vi "Set and Measure VSEC.vi"(4 "Header":string="HighVsec", 6 "Name":string, 7 "Position in":u32, 8 "error in (no error)":errorcluster, 9 "Measurement Wait Time":u32, 10 "Cree Comms in":refnum<class "Cree Communications.lvclass">, 11 "Calibration in":refnum<class "Calibration.lvclass">) -> (0 "error out":errorcluster, 2 "DSpic Measurement":dbl, 3 "Actual Measurement":dbl)   [LabVIEW 2015, in "Calibration.lvclass"]
uses:
  Calibration.lvclass
  Classes/Cree Communications/Class/Cree Communications.lvclass
  Classes/Cree Communications/Cree Comms Messages/Set Vsec/Set Vsec Reference.lvclass
  Classes/Cree Communications/Cree Comms Messages/CC Message/CC Message.lvclass/CC Message.ctl
  Test Class/Test Class.lvclass
  Classes/Cree Communications/Cree Comms Messages/CC Message/CC Message.lvclass
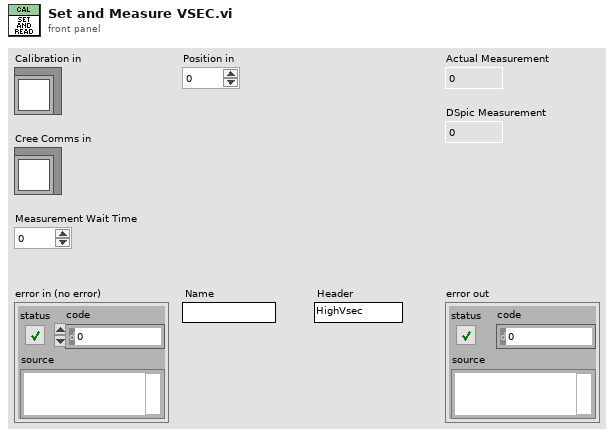
[diagram p1: front panel]
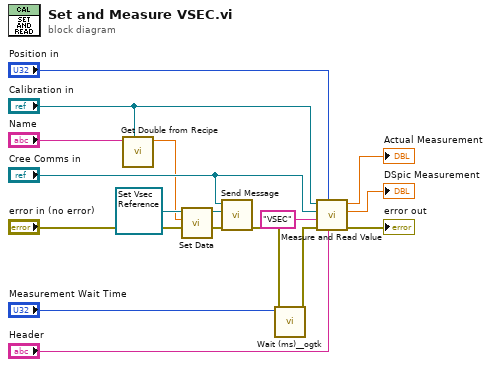
[diagram p0: block diagram]
diagram:
  n1 = call "Get Double from Recipe.vi"("Test Class in"="Calibration in", "Name"="Name") -> ("Value"=w7:dbl)  [unwired: 7 in, 2 out]
  n2 = call "Set Data.vi"("Data"=w7, "CC Message in"=refnum<class "Set Vsec Reference.lvclass"> refnum ("Cree Comms Messages.lvlib:Set Vsec.lvclass")) -> ("CC Message out"=w6:refnum<class "Set Vsec Reference.lvclass">)  [unwired: 8 in, 1 out]
  n3 = call "Send Message.vi"("error in (no error)"="error in (no error)", "Cree Comms Message"=w6, "Acrobat Template in"="Cree Comms in") -> ("error out"=w10:errorcluster)  [unwired: 7 in, 1 out]
  n4 = call <userlib>:"Wait (ms)__ogtk.vi"("error in (no error)"=w10, "milliseconds to wait"="Measurement Wait Time") -> ("error out"=w11:errorcluster)  [unwired: 8 in, 1 out]
  n5 = call "Measure and Read Value.vi"("Header"="Header", "Position"="Position in", "error in (no error)"=w11, "Calibration Type"="VSEC", "Cree Communications"="Cree Comms in", "Calibration in"="Calibration in") -> ("error out"=→"error out":errorcluster, "DSpic Measurement"=→"DSpic Measurement":dbl, "Actual Measurement"=→"Actual Measurement":dbl)  [unwired: 3 in]
